vi "Quadrature Integrand.vi"(10 "data":variant, 11 "X":dbl[](array[numeric])) -> (0 "error out":errorcluster, 3 "F(X)":dbl[](array[numeric]))   [LabVIEW 2023]
doc: "This VI calculates the integrand function F(X)."
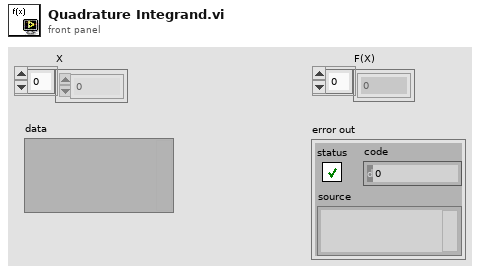
[diagram p1: front panel]
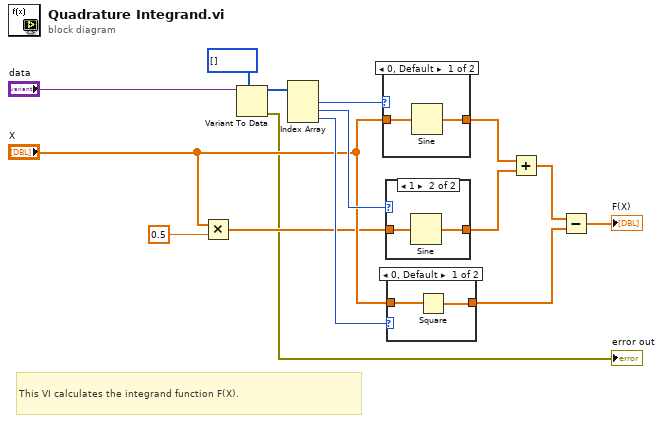
[diagram p0: block diagram]
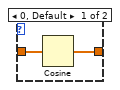
[diagram p3: hidden frame]
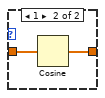
[diagram p4: hidden frame]
diagram:
  # "This VI calculates the integrand function F(X)."
  n1 = Multiply(x="X", y=0.5) -> (x*y=w7:dbl[])
  n2 = Variant To Data(type=u16[] [], Variant="data") -> (data=w12:u16[], error out=→"error out":errorcluster)  [unwired: 1 in]
  n3 = Index Array(array=w12) -> (element #1=w11:u16, element #2=w10:u16, element #3=w9:u16)  [unwired: 3 in]
  n4 = case shown="0, Default" w11 {
    tunnel: "X" -> [w17 w19]
    tunnel: [w16 w18] -> w6
    frame 0, Default {
      n5 = Sine(x=w17) -> (sin(x)=w16:dbl[])
    }
    frame 1 {
      n6 = Cosine(x=w19) -> (cos(x)=w18:dbl[])
    }
  }
  n7 = case shown="1" w10 {
    tunnel: w7 -> [w21 w22]
    tunnel: [w20 w23] -> w5
    frame 0, Default {
      n8 = Cosine(x=w21) -> (cos(x)=w20:dbl[])
    }
    frame 1 {
      n9 = Sine(x=w22) -> (sin(x)=w23:dbl[])
    }
  }
  n10 = case shown="0, Default" w9 {
    tunnel: "X" -> [w25 w26]
    tunnel: [w24 w26] -> w3
    frame 0, Default {
      n11 = Square(x=w25) -> (x^2=w24:dbl[])
    }
    frame 1 {
    }
  }
  n12 = Add(x=w6, y=w5) -> (x+y=w4:dbl[])
  n13 = Subtract(x=w4, y=w3) -> (x-y=→"F(X)":dbl[])
